vi "XYStage.WriteAcceleration(real).vi"(8 "error in (no error)":errorcluster, 10 "Acceleration (units/s^2)":dbl, 11 "XYStage in":refnum<class "XYStage.lvclass">) -> (0 "error out":errorcluster, 2 "Acceleration (counts/s^2)":i32, 3 "XYStage out":refnum<class "XYStage.lvclass">)   [LabVIEW 2019, in "XYStage.lvclass"]
uses:
  XYStage.lvclass
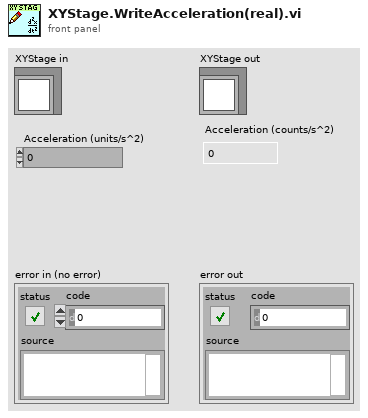
[diagram p1: front panel]
types:
  T1 = typedef "XYStage.lvclass/PrivateData--Ref.ctl" = refnum<data-value>
  T2 = typedef "XYStage.lvclass/PrivateData--Cluster.ctl" = cluster{"Dependencies":T3, "Public Events":T4, "Protected Events":T5, "Private Events":T6, "Configuration":T7, "Target":T8, "Move Parameters":T11}
  T3 = typedef "XYStage.lvclass/Dependencies--Cluster.ctl" = cluster{"Positions":refnum<class "SMO.Dictionary.Variant.lvclass">}
  T4 = typedef "XYStage.lvclass/PublicEvents--Cluster.ctl" = cluster{"MoveComplete":refnum<user-event>, "NewPosition":refnum<user-event>, "UpdatedNamedPosition":refnum<user-event>, "MoveStarted":refnum<user-event>}
  T5 = typedef "XYStage.lvclass/ProtectedEvents--Cluster.ctl" = cluster{"API_Template":refnum<user-event>}
  T6 = typedef "XYStage.lvclass/PrivateEvents--Cluster.ctl" = cluster{"MoveAbsolute":refnum<user-event>, "MoveRelative":refnum<user-event>, "MoveToNamedPosition":refnum<user-event>, "StorePosition":refnum<user-event>, "Home":refnum<user-event>}
  T7 = typedef "XYStage.lvclass/Configuration--Cluster.ctl" = cluster{"Real-World Units":string, "Counts per Unit":dbl}
  T8 = typedef "XYStage.lvclass/TargetPositions--Cluster.ctl" = cluster{"Coords":T9, "Counts":T10}
  T9 = typedef "XYStage.lvclass/(real)Coords--Cluster.ctl" = cluster{"X":dbl, "Y":dbl}
  T10 = typedef "XYStage.lvclass/(counts)Coords--Cluster.ctl" = cluster{"X":i32, "Y":i32}
  T11 = typedef "XYStage.lvclass/MoveParameters--Cluster.ctl" = cluster{"Velocity (units/s)":dbl, "Acceleration (units/s^2)":dbl}
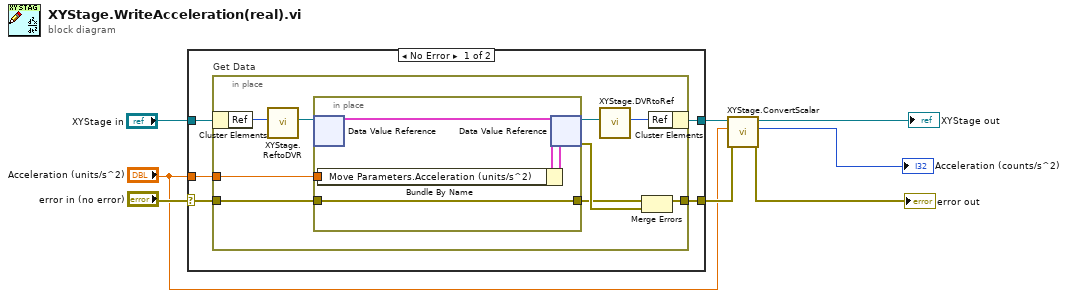
[diagram p0: block diagram]
diagram:
  n1 = case shown="No Error" "error in (no error)" {
    selector: "error in (no error)" -> [w12 w27]
    tunnel: "XYStage in" -> [w13 w28]
    tunnel: [w10 w27] -> w4
    tunnel: [w11 w28] -> w6
    tunnel: "Acceleration (units/s^2)" -> [w9 _]
    frame No Error {
      n2 = in-place "Get Data" {
        in-place-border: w12 -> [w22]
        in-place-border: [w19] -> w10
        in-place-border: w9 -> [w14]
        n3 = in-place-cluster #1(w13) -> ("Ref"=w18:u32)
        n4 = call "XYStage.ReftoDVR.vi"("Ref"=w18) -> ("Ref"=w16:T1)  [unwired: 10 in]
        n5 = in-place {
          in-place-border: w22 -> [w26]
          in-place-border: [w26] -> w20
          in-place-border: w14 -> [w24]
          n6 = in-place-dvr #2(w16) -> (w23:T2)  [unwired: 1 out]
          n7 = Bundle By Name(cluster=w23, "Move Parameters.Acceleration (units/s^2)"=w24) -> (w25:T2)
          n8 = in-place-dvr #2(w25) -> (w17:T1, w21:errorcluster)
        }
        n9 = call "XYStage.DVRtoRef.vi"("Ref"=w17) -> ("Ref"=w15:u32)  [unwired: 10 in]
        n10 = Merge Errors(w20, w21) -> (w19:errorcluster)
        n11 = in-place-cluster #1("Ref"=w15) -> (w11:refnum<class "XYStage.lvclass">)
      }
    }
    frame Error {
    }
  }
  n12 = call-dynamic "XYStage.ConvertScalar.vi"("error in (no error)"=w4, "Units"="Acceleration (units/s^2)", "XYStage in"=w6) -> ("error out"=→"error out":errorcluster, "Counts out"=→"Acceleration (counts/s^2)":i32, "XYStage out"=→"XYStage out":refnum<class "XYStage.lvclass">)  [unwired: 5 in, 1 out]
